vi "NTC R2T_regi.vi"(8 "C=":dbl=1.53701e-07, 9 "B=":dbl=0.000261679, 10 "A=":dbl=0.00129231, 11 "R [Ohm]":dbl) -> (3 "T [°C]":dbl)   [LabVIEW 2014]
panel:
  # "--->"
  # "A default értékek 2k-s\nNTC-re vonatkoznak."
  # "Steinhart-Hart egyenlet: \n1/T[K]=A+B*ln(R[Ohm])+C*(ln(R[Ohm))^3"
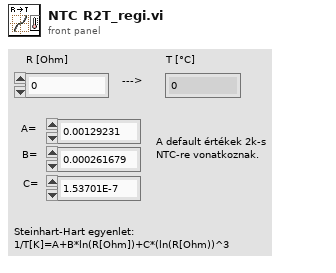
[diagram p1: front panel]
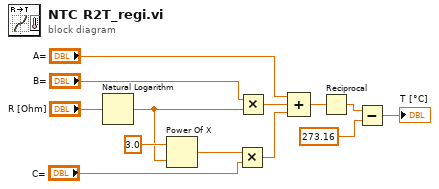
[diagram p0: block diagram]
diagram:
  n1 = Natural Logarithm(1:"R [Ohm]") -> (0:w9:dbl)
  n2 = Power Of X(1:w9, 2:3.0 ("element")) -> (0:w8:dbl)
  n3 = Multiply(x=w8, y="C=") -> (x*y=w5:dbl)
  n4 = Multiply(x="B=", y=w9) -> (x*y=w6:dbl)
  n5 = Compound Arithmetic op=ADD("A=", w6, w5) -> (w4:dbl)
  n6 = Reciprocal(x=w4) -> (1/x=w3:dbl)
  n7 = Subtract(x=w3, y=273.16) -> (x-y=→"T [°C]":dbl)
